vi "Measure.vi"(8 "Error In":errorcluster, 11 "reference in":refnum<class "ByRef1.lvclass">) -> (0 "Error Out":errorcluster, 2 "Measurement":dbl, 3 "reference out":refnum<class "ByRef1.lvclass">)   [LabVIEW 2020, in "ByRef1.lvclass"]
uses:
  ByRef1.lvclass
  57184dfa-e3d9-4e6c-83a8-a13ee8c92110.vi
  <vilib>/Analysis/NI_AALBase.lvlib
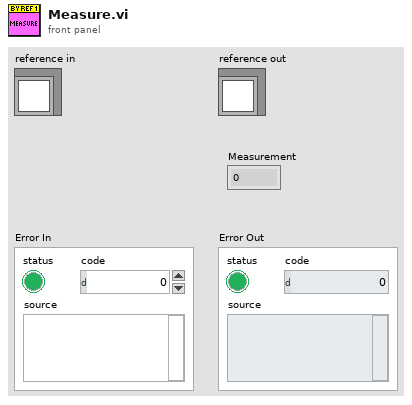
[diagram p1: front panel]
types:
  T1 = typedef "ByRef1.lvclass/ObjectAttributes.ctl" = cluster{"Triggers":i32}
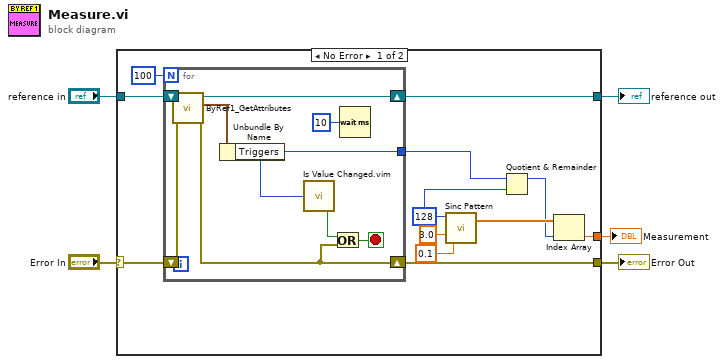
[diagram p0: block diagram]
diagram:
  n1 = case shown="No Error" "Error In" {
    selector: "Error In" -> [w17 w28]
    tunnel: [w16 w28] -> w4
    tunnel: [w14 w27] -> w2
    tunnel: "reference in" -> [w15 w27]
    tunnel: [w8 _] -> w1
    frame No Error {
      w11 = 128 ("samples")
      n2 = for {
        N: 100 -> [_]
        shift-right: [w21] -> w16
        shift-left: w17 -> [w26]
        shift-right: [w23] -> w14
        shift-left: w15 -> [w24]
        tunnel: [w18] -> w12
        stop <- w19 stop-if-true
        n3 = call "ByRef1_GetAttributes.vi"("error in (no error)"=w26, "reference in"=w24) -> ("error out"=w21:errorcluster, "Data"=w25:T1, "reference out"=w23:refnum<class "ByRef1.lvclass">)  [unwired: 6 in, 1 out]
        n4 = Unbundle By Name(w25) -> ("Triggers"=w18:i32)
        n5 = call "Is Value Changed.vim"("value"=w18) -> ("changed or first call?"=w20:bool)
        n6 = Or(x=w20, y=w21) -> (x .or. y?=w19:bool)
        n7 = Wait (ms)(milliseconds to wait=u32 10) -> ()  [unwired: 1 out]
      }
      n8 = call <vilib>:"Sinc Pattern.vi"("delta t"=0.1, "delay"=3.0, "samples"=w11) -> ("Sinc Pattern"=w10:dbl[])  [unwired: 1 in, 1 out]
      n9 = Quotient & Remainder(x=w12, y=w11) -> (x-y*floor(x/y)=w9:i32)  [unwired: 1 out]
      n10 = Index Array(array=w10, index=w9) -> (element=w8:dbl)
    }
    frame Error {
    }
  }
  "Error Out" <- w4
  "reference out" <- w2
  "Measurement" <- w1
